vi "Server.vi"() -> ()   [LabVIEW 2021]
panel:
  out "XY Graph":cluster{dbl[], dbl[]}(graph)
  out "Client_IP":string
  in  "stop":bool
  out "Frame_OK":bool
  out "Recieved_Frames":u16
  out "Client_ID":u8
  out "Recieved frame_after_error_checks":T1
  out "Recieved_Frame_fails_the_check":bool
  out "error out":errorcluster
  out "Remote port":u16
  out "remote address":string
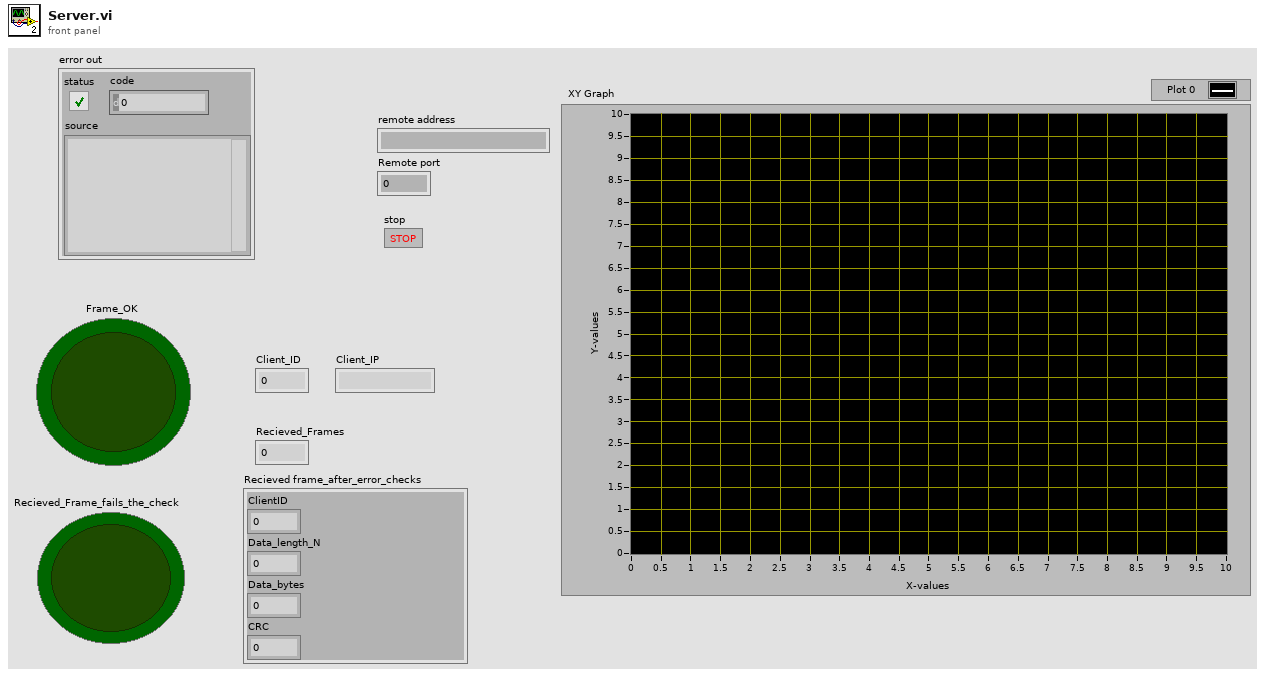
[diagram p1: front panel]
types:
  T1 = cluster{"ClientID":u8, "Data_length_N":i32, "Data_bytes":u8, "CRC":u8}
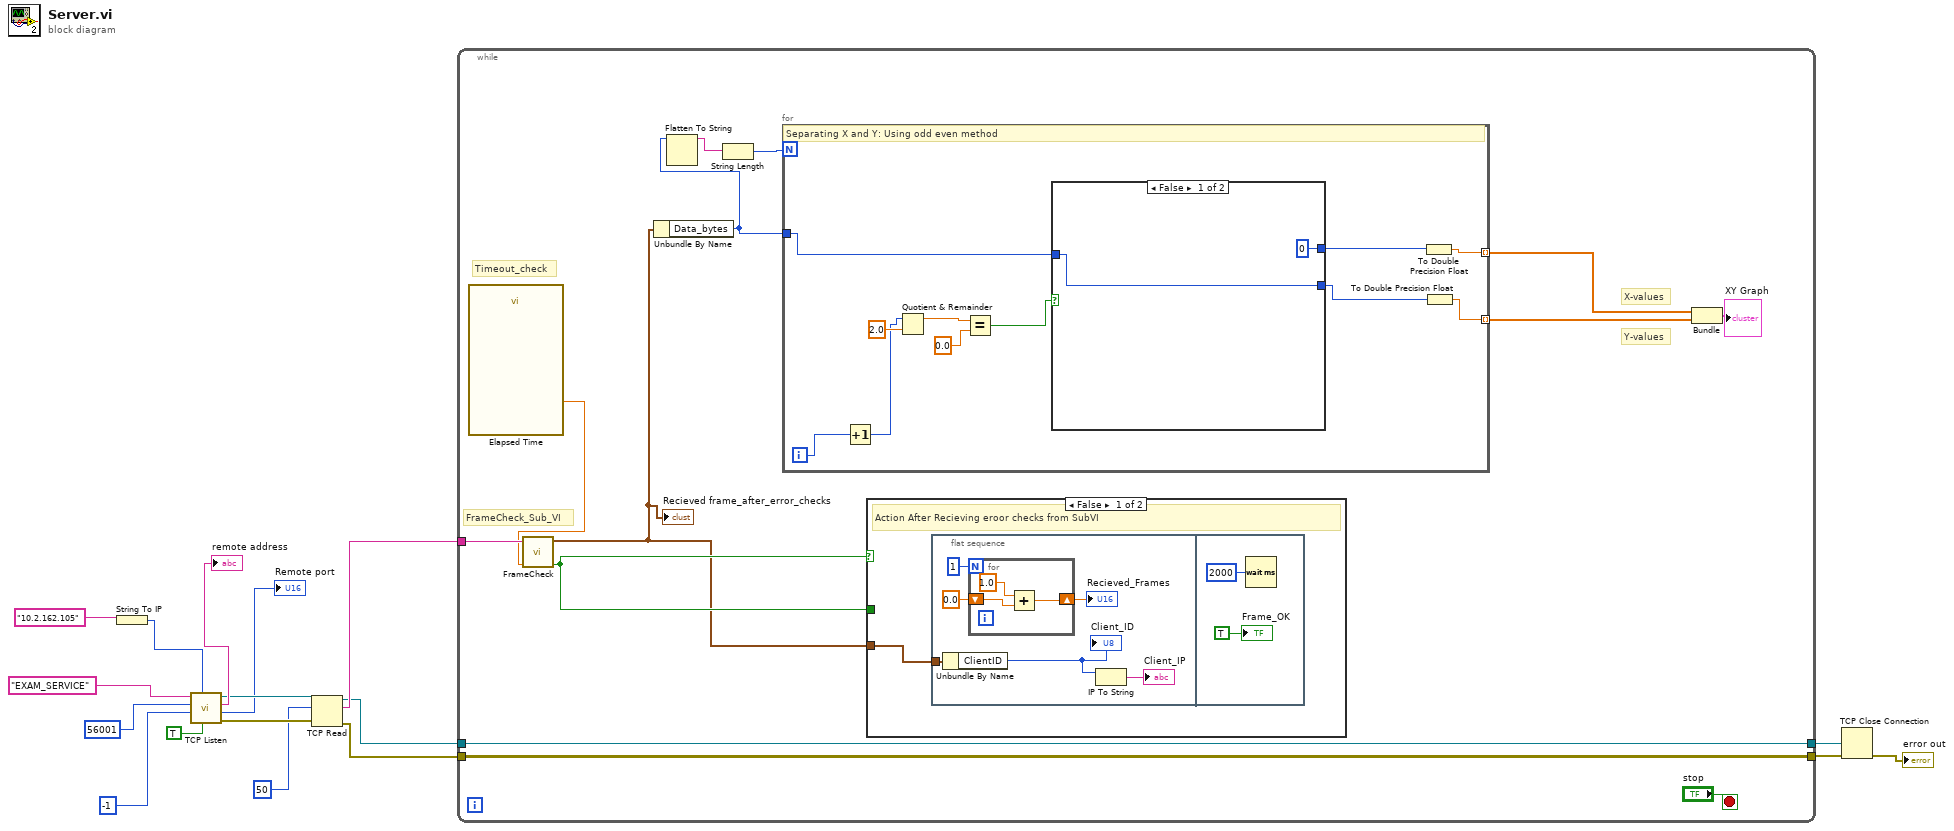
[diagram p0: block diagram]
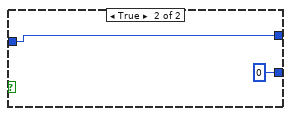
[diagram p2: hidden frame]
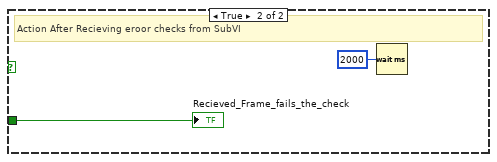
[diagram p3: hidden frame]
diagram:
  n1 = String To IP(1:"10.2.162.105") -> (0:w9:u32)
  n2 = call <vilib>:"TCP Listen.vi"("resolve remote address (T)"=TRUE, "net address"=w9, "timeout ms (wait forever: -1)"=-1, "port"=u16 56001, "service name"="EXAM_SERVICE") -> ("error out"=w13:errorcluster, "remote port"=→"Remote port":u16, "remote address"=→"remote address":string, "connection ID"=w12:refnum<k5>)  [unwired: 2 in, 1 out]
  n3 = TCP Read(connection ID=w12, bytes to read=50, error in (no error)=w13) -> (connection ID out=w2:refnum<k5>, data out=w5:string, error out=w4:errorcluster)  [unwired: 2 in]
  n4 = while {
    tunnel: w5 -> [w30]
    tunnel: [w28] -> w3
    tunnel: w4 -> [w28]
    tunnel: w2 -> [w27]
    tunnel: [w27] -> w1
    stop <- "stop" stop-if-true
    # "Timeout_check"
    # "X-values"
    # "Y-values"
    # "FrameCheck_Sub_VI"
    n5 = call "Elapsed Time"() -> ("Elapsed Time (s)"=w18:dbl)  [unwired: 12 in, 7 out]
    n6 = call "FrameCheck.vi"("Timeout_Indicator"=w18, "Recieved_string_SingleFrame"=w30) -> ("Recieved_Frame_fails_the_check"=w29:bool, "Recieved frame_after_error_checks"=w26:T1)  [unwired: 8 in]
    "Recieved frame_after_error_checks" <- w26
    n7 = Unbundle By Name(w26) -> ("Data_bytes"=w23:u8)
    n8 = Flatten To String(anything=w23) -> (data string=w25:string)  [unwired: 3 in, 2 out]
    n9 = String Length(string=w25) -> (length=w24:i32)
    n10 = for {
      N: w24 -> [_]
      tunnel: w23 -> [w37]
      tunnel: [w32] -> w21 mode=indexing
      tunnel: [w31] -> w20 mode=indexing
      i -> [w36]
      # "Separating X and Y: Using odd even method"
      n11 = Increment(x=w36) -> (x+1=w35:i32)
      n12 = Quotient & Remainder(x=w35, y=2.0) -> (x-y*floor(x/y)=w41:dbl)  [unwired: 1 out]
      n13 = Equal?(x=w41, y=0.0) -> (x = y?=w38:bool)
      n14 = case shown="False" w38 {
        tunnel: [u8 0 ("Data_bytes") w44] -> w33
        tunnel: w37 -> [w43 w44]
        tunnel: [w43 u8 0 ("Data_bytes")] -> w34
        frame False {
        }
        frame True {
        }
      }
      n15 = To Double Precision Float(number=w33) -> (double precision float=w32:dbl)
      n16 = To Double Precision Float(number=w34) -> (double precision float=w31:dbl)
    }
    n17 = case shown="False" w29 {
      tunnel: w26 -> [w46 _]
      tunnel: w29 -> [_ w59]
      frame False {
        # "Action After Recieving eroor checks from SubVI"
        n18 = flat-sequence {
          tunnel: w46 -> [w50]
          frame #0 {
            n19 = Unbundle By Name(w50) -> ("ClientID"=w49:u8)
            "Client_ID" <- w49
            n20 = for {
              N: 1 -> [_]
              shift-right: [w54] -> w52
              shift-left: 0.0 -> [w53]
              n21 = Add(x=1.0, y=w53) -> (x+y=w54:dbl)
            }
            "Recieved_Frames" <- w52
            n22 = IP To String(2:w49) -> (0:→"Client_IP":string)  [unwired: 1 in]
          }
          frame #1 {
            n23 = Wait (ms)(milliseconds to wait=u32 2000) -> ()  [unwired: 1 out]
            "Frame_OK" <- TRUE ("Frame_OK")
          }
        }
      }
      frame True {
        # "Action After Recieving eroor checks from SubVI"
        n24 = Wait (ms)(milliseconds to wait=u32 2000) -> ()  [unwired: 1 out]
        "Recieved_Frame_fails_the_check" <- w59
      }
    }
    n25 = Bundle(w21, w20) -> (→"XY Graph":cluster{dbl[], dbl[]})  [unwired: 1 in]
  }
  n26 = TCP Close Connection(connection ID=w1, error in (no error)=w3) -> (error out=→"error out":errorcluster)  [unwired: 1 in, 1 out]
